vi "niRFUtil CONV 1 Ohm Voltage to 1 Ohm Watt (real wfm).vi"(7 "Real Waveform (V)":T1 {"y" min=0 max=127 format="%.2f"; "dx" format="%^.2e"; "x0" format="%^.2e"}) -> (8 "Real Waveform (W)":T1 {"y" min=0 max=127 format="%.2f"; "dx" format="%^.2e"; "x0" format="%^.2e"})   [LabVIEW 2015, in "niRFUtil.lvlib"]
doc: "(c) Copyright 2006, National Instruments, Inc. This VI may not be duplicated, sold, or distributed without written consent from National Instruments."
uses:
  niRFUtil.lvlib
  Includes/niRFUtil INC Real Waveform.ctl
  Includes/niRFUtil INC Real Array.ctl
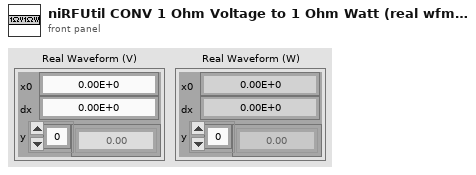
[diagram p1: front panel]
types:
  T1 = typedef "niRFUtil.lvlib/niRFUtil INC Real Waveform.ctl" = cluster{"x0":dbl, "dx":dbl, "y":T2}
  T2 = typedef "niRFUtil.lvlib/niRFUtil INC Real Array.ctl" = sgl[]
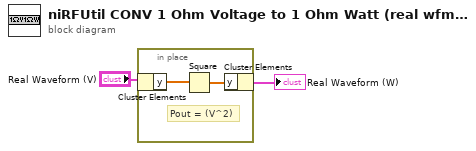
[diagram p0: block diagram]
diagram:
  n1 = in-place {
    # "Pout = (V^2)"
    n2 = in-place-cluster #1("Real Waveform (V)") -> ("y"=w4:T2)
    n3 = Square(x=w4) -> (x^2=w3:T2)
    n4 = in-place-cluster #1("y"=w3) -> (→"Real Waveform (W)":T1)
  }
